vi "SwitchingHTTPCameraResponder.vi"(9 "Switched Camera Name":string, 10 "parameters":T1(array[cluster]), 11 "connection ID":refnum<k5>) -> ()   [LabVIEW 2017, in "ArgosLib.lvlib"]
doc: "This VI is launched each time a new client camera connection is requested. The connection will remain open until closed by the client or because of errors with the camera. Parameters are name/lvalue pairs that have been parsed from a URL request. Supported parameters are name, fps, resolution, compression, exposure, brightness, whitebalance, sharpness, and colorlevel.\n\nThe first four parameters are filled with defaults if not provided, but the latter four are only set if provided."
uses:
  <vilib>/Rock Robotics/SystemInterfaces/NetworkCommunication/NetComm_UsageReport_ResourceType.ctl
  <vilib>/Rock Robotics/WPI/Camera/WPI_CameraImageSize.ctl
  PowerUpSrc/Global_Var-RefNum/SwitchedCameraData.vi
  <vilib>/Utility/error.llb/Error Cluster From Error Code.vi
  <vilib>/ErrorRing/Error Ring.xnode
  ArgosLib.lvlib
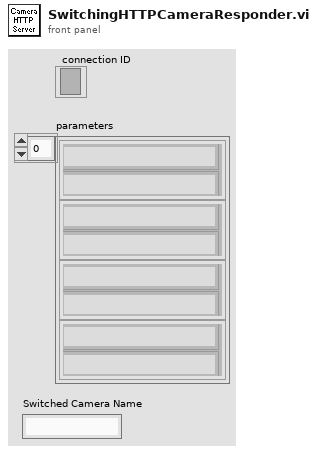
[diagram p1: front panel]
types:
  T1 = cluster{"token string":string, "token string 2":string}[]
  T2 = typedef "Image Type" = u32
  T3 = cluster{"White Balance":string, "Brightness":i32, "Sharpness":i32, "Saturation":i32, "Exposure":string}
  T4 = cluster{"Camera Name":string, "Size":string, "Frame Rate":i32, "Compression":i32}
  T5 = typedef "NetComm_UsageReport_ResourceType.ctl" = enum8{"Controller", "Module", "Language", "CANPlugin", "Accelerometer", "ADXL345", "AnalogChannel", "AnalogTrigger", "AnalogTriggerOutput", "CANJaguar", "Compressor", "Counter", "Dashboard", "DigitalInput", "DigitalOutput", "DriverStationCIO", "DriverStationEIO", "DriverStationLCD", "Encoder", "GearTooth", "Gyro", "I2C", "Framework", "Jaguar", "Joystick", "Kinect", "KinectStick", "PIDController", "Preferences", "PWM", "Relay", "RobotDrive", "SerialPort", "Servo", "Solenoid", "SPI", "Task", "Ultrasonic", "Victor", "Button", "Command", "AxisCamera", "PCVideoServer", "SmartDashboard", "Talon", "HiTechnicColorSensor", "HiTechnicAccel", "HiTechnicCompass", "SRF08", "AnalogOutput", "Victor SP", "Talon SRX", "CAN Talon SRX", "ADXL362 Accel", "ADXRS450 Gyro", "Rev SPARK", "Mindsensors SD540", "Digital Filter", "ADIS16448", "PDP", "PCM", "PigeonIMU", "Nidec Brushless", "CTRE CANifier", "CTRE Future 0", "CTRE Future 1", "CTRE Future 2", "CTRE Future 3", "CTRE Future 4", "CTRE Future 5", "CTRE Future 6"}
  T6 = cluster{"White Balance":bool, "Brightness":bool, "Sharpness":bool, "Saturation":bool, "Exposure":bool}
  T7 = typedef "IMAQ Image.ctl" = refnum<image>
  T8 = typedef "WPI_CameraImageSize.ctl" = enum16{"640x480", "320x240", "160x120", "Custom"}
  T9 = enum16{"Update Mode", "Get Image", "Get Image Data"}
  T10 = typedef "WPI_CameraDevRef.ctl" = cluster{"Camera Address":string, "CameraStatus":errorcluster}
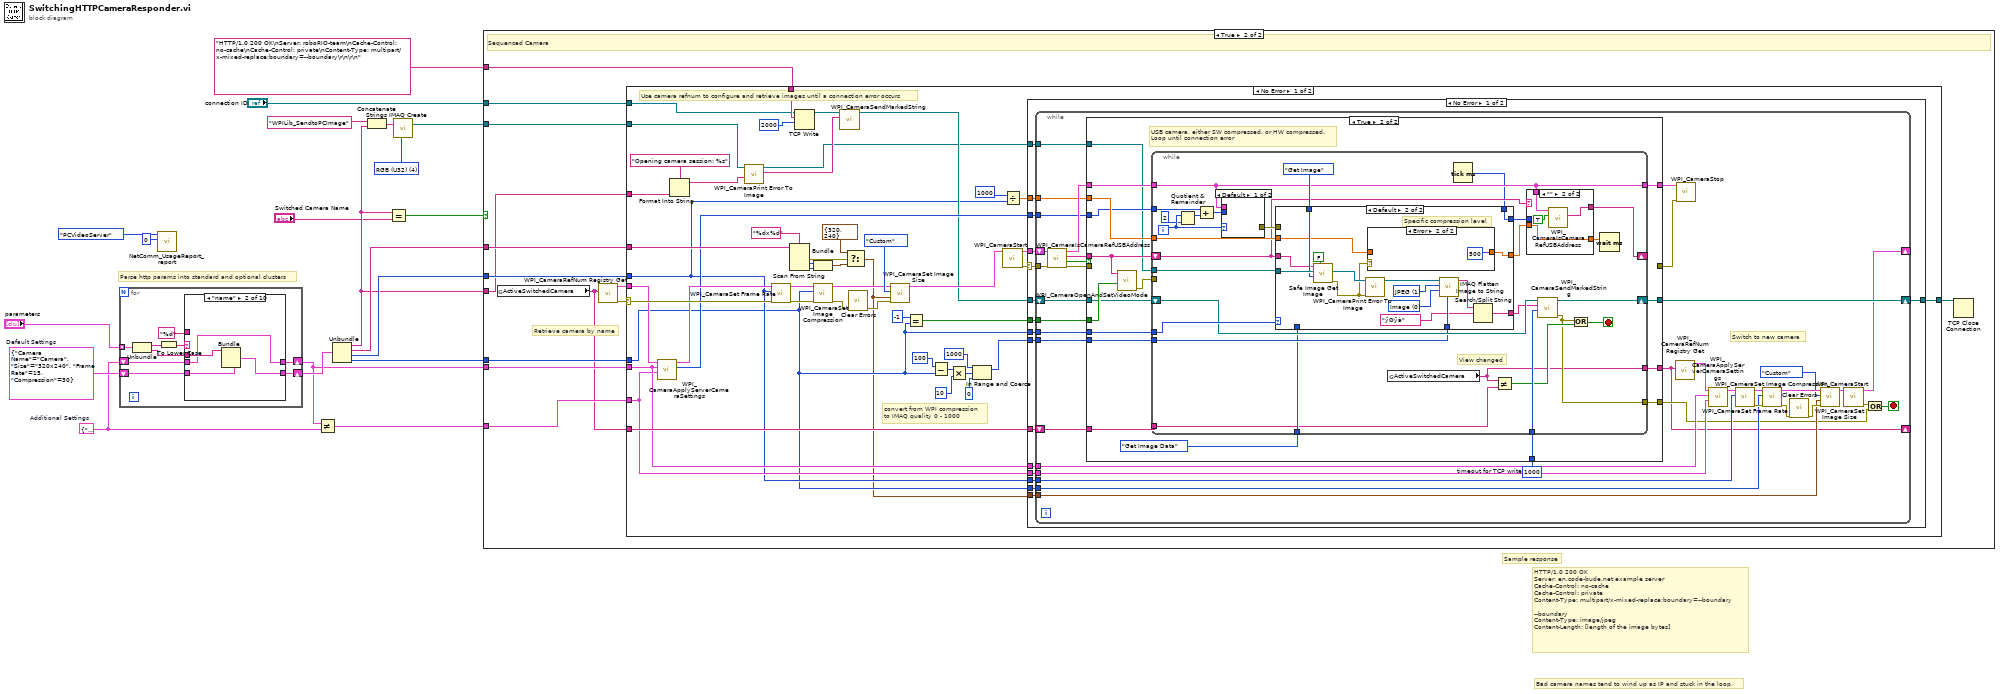
[diagram p0: block diagram]
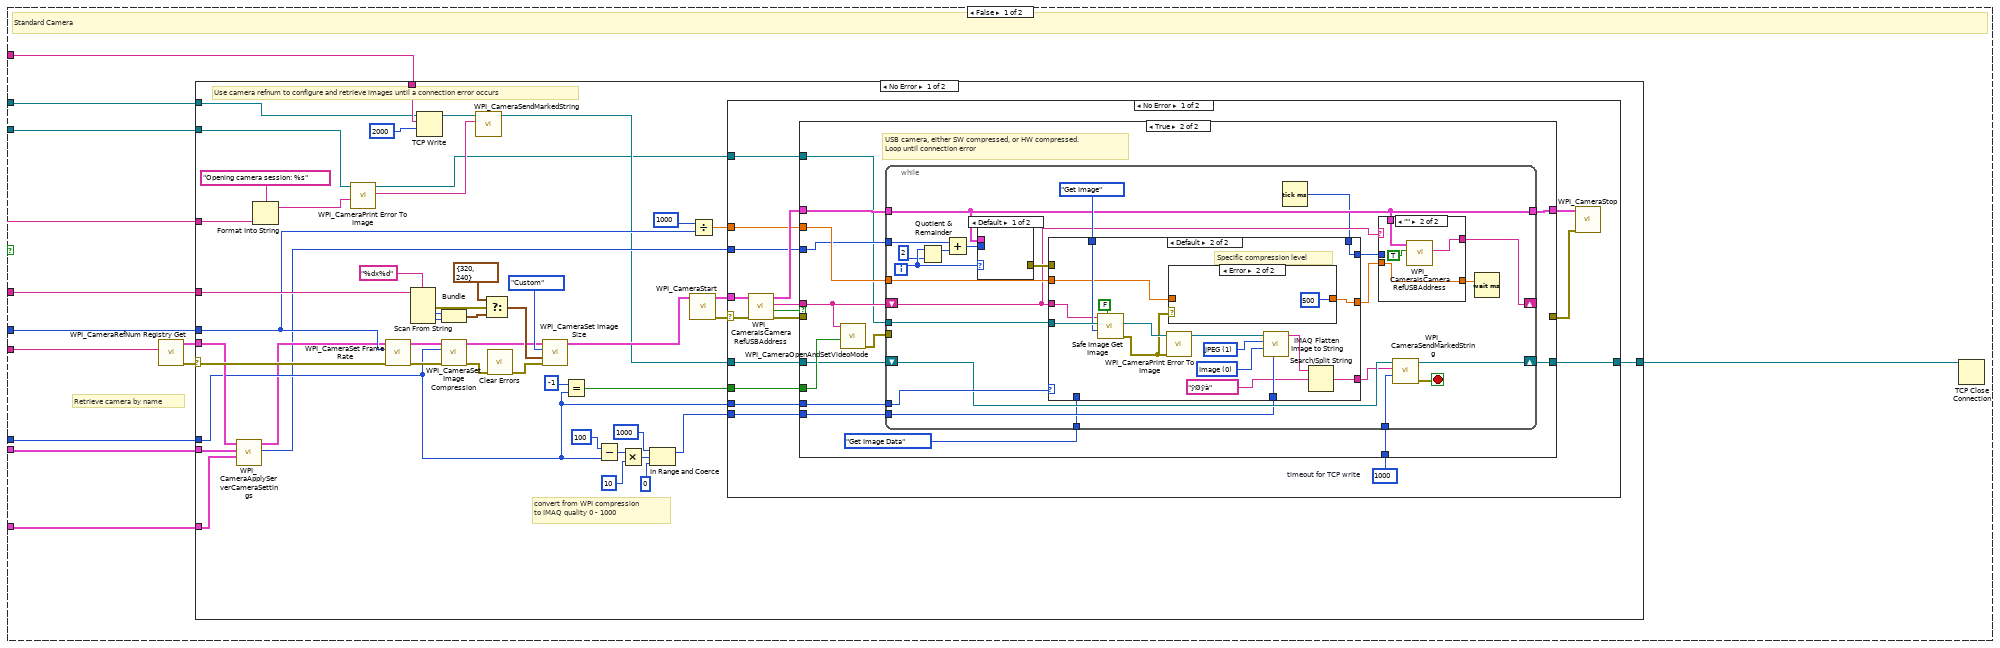
[diagram p2: hidden frame]
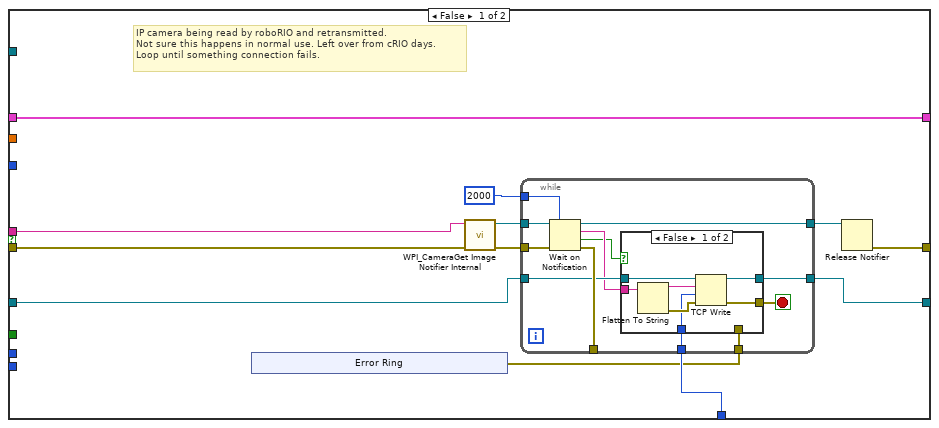
[diagram p3: hidden frame]
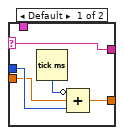
[diagram p5: hidden frame]
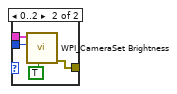
[diagram p6: hidden frame]
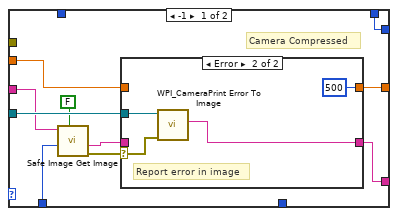
[diagram p7: hidden frame]
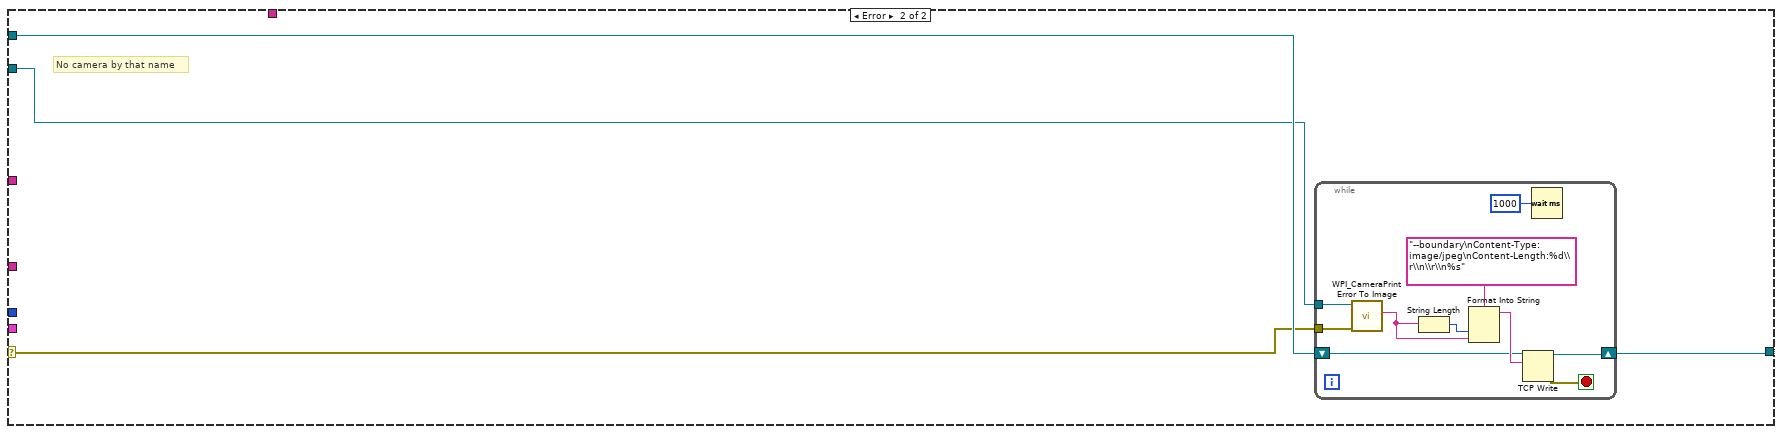
[diagram p11: hidden frame]
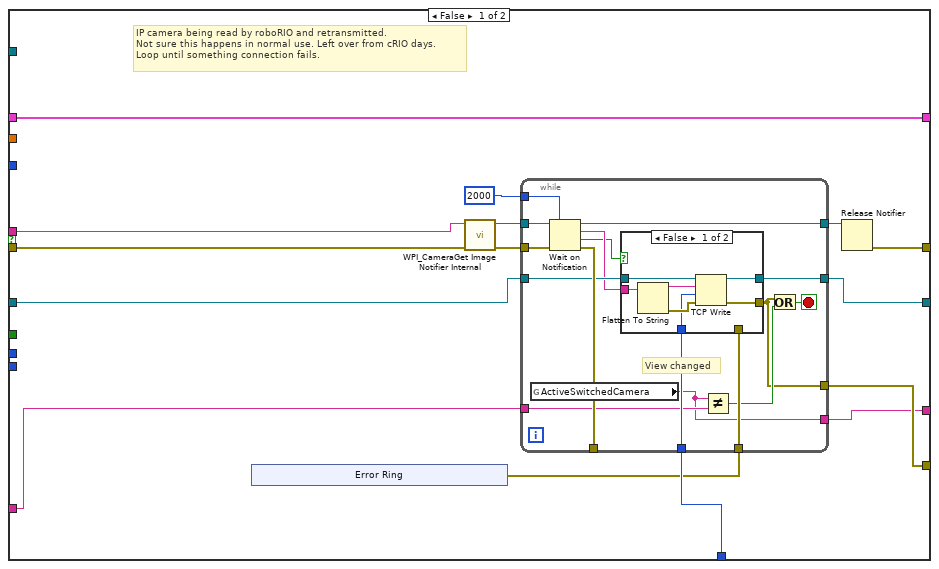
[diagram p12: hidden frame]
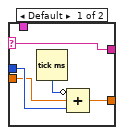
[diagram p14: hidden frame]
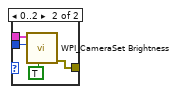
[diagram p15: hidden frame]
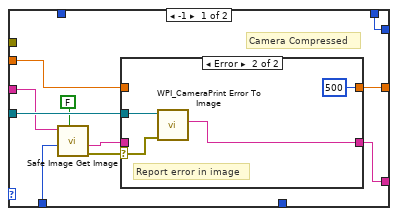
[diagram p16: hidden frame]
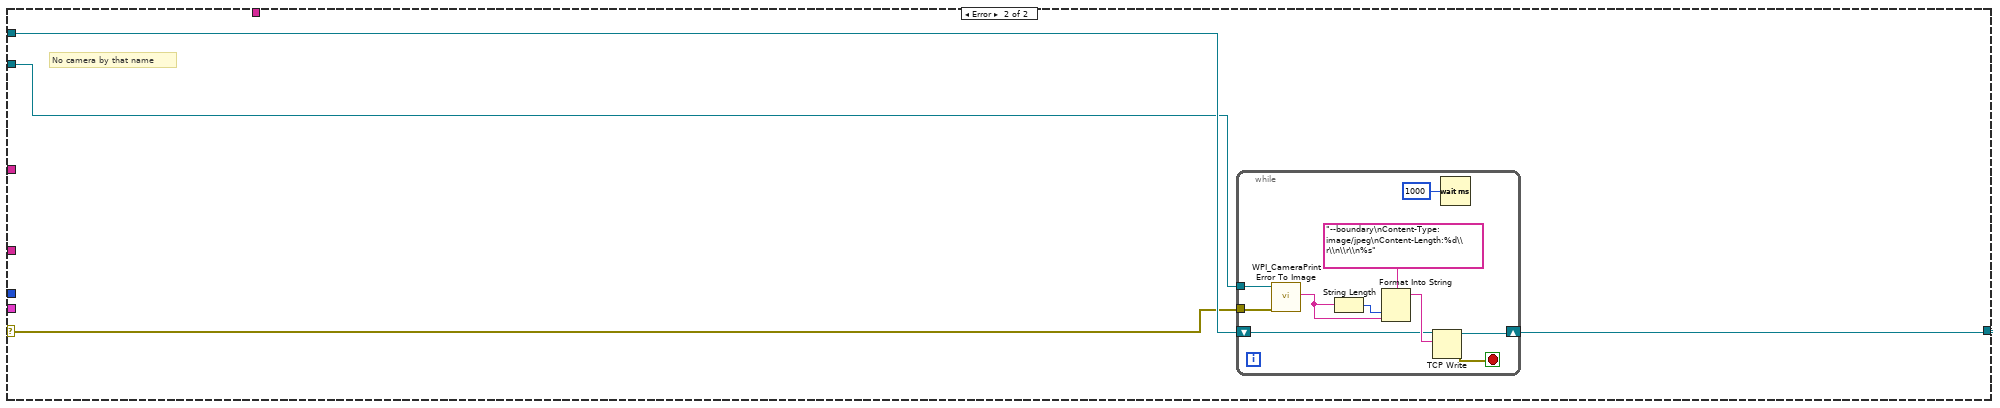
[diagram p20: hidden frame]
diagram:
  w6 = T2 4 items=["Grayscale (U8)", "Grayscale (I16)", "Grayscale (SGL)", "Complex (CSG)", "RGB (U32)", "HSL (U32)", "RGB (U64)", "Grayscale (U16)"] ("Image Type")
  w13 = T3 {"White Balance"="", "Brightness"=-1, "Sharpness"=-1, "Saturation"=-1, "Exposure"=""}  # Additional Settings
  w18 = T4 {"Camera Name"="Camera", "Size"="320x240", "Frame Rate"=15, "Compression"=30}  # Default Settings
  # "Sample response"
  # "HTTP/1.0 200 OK\nServer: en.code-bude.net example server\nCache-Control: no-cache\nCache-Control: private\nContent-Type: multipart/x-mixed-replace;boundary=--boundary\n \n--boundary\nContent-Type: image/jpeg\nContent-Length: [length of the image bytes]"
  # "Parse http params into standard and optional clusters"
  # "Bad camera names tend to wind up as IP and stuck in the loop."
  n1 = for {
    tunnel: "parameters" -> [w29] mode=indexing
    shift-right: [w24] -> w16
    shift-left: w18 -> [w26]
    shift-right: [w21] -> w11
    shift-left: w13 -> [w22]
    n2 = Unbundle(w29) -> ("token string"=w28:string, "token string 2"=w25:string)
    n3 = To Lower Case(string=w28) -> (all lower case string=w27:string)
    n4 = case shown="\"name\"" w27 {
      tunnel: w26 -> [w31 w35 w41 w45 w51 w55 w59 w65 w71 w77]
      tunnel: w25 -> [_ w34 w39 w43 w49 w53 w56 w61 w67 w73]
      tunnel: [w31 w33 w40 w44 w50 w55 w59 w65 w71 w77] -> w24
      tunnel: "%d" -> [_ _ w38 _ w47 _ _ w62 w68 w74]
      tunnel: w22 -> [w30 w32 w36 w42 w46 w54 w58 w64 w70 w76]
      tunnel: [w30 w32 w36 w42 w46 w52 w57 w63 w69 w75] -> w21
      frame Default {
      }
      frame "name" {
        n5 = Bundle(cluster=w35, "Camera Name"=w34) -> (w33:T4)  [unwired: 3 in]
      }
      frame "fps" {
        n6 = Scan From String(format string=w38, input string=w39) -> (output 1=w37:i32)  [unwired: 3 in, 3 out]
        n7 = Bundle(cluster=w41, "Frame Rate"=w37) -> (w40:T4)  [unwired: 3 in]
      }
      frame "resolution" {
        n8 = Bundle(cluster=w45, "Size"=w43) -> (w44:T4)  [unwired: 3 in]
      }
      frame "compression" {
        n9 = Scan From String(format string=w47, input string=w49) -> (output 1=w48:i32)  [unwired: 3 in, 3 out]
        n10 = Bundle(cluster=w51, "Compression"=w48) -> (w50:T4)  [unwired: 3 in]
      }
      frame "whitebalance" {
        n11 = Bundle(cluster=w54, "White Balance"=w53) -> (w52:T3)  [unwired: 4 in]
      }
      frame "exposure" {
        n12 = Bundle(cluster=w58, "Exposure"=w56) -> (w57:T3)  [unwired: 4 in]
      }
      frame "brightness" {
        n13 = Scan From String(format string=w62, input string=w61) -> (output 1=w60:i32)  [unwired: 3 in, 3 out]
        n14 = Bundle(cluster=w64, "Brightness"=w60) -> (w63:T3)  [unwired: 4 in]
      }
      frame "sharpness" {
        n15 = Scan From String(format string=w68, input string=w67) -> (output 1=w66:i32)  [unwired: 3 in, 3 out]
        n16 = Bundle(cluster=w70, "Sharpness"=w66) -> (w69:T3)  [unwired: 4 in]
      }
      frame "colorlevel" {
        n17 = Scan From String(format string=w74, input string=w73) -> (output 1=w72:i32)  [unwired: 3 in, 3 out]
        n18 = Bundle(cluster=w76, "Saturation"=w72) -> (w75:T3)  [unwired: 4 in]
      }
    }
  }
  n19 = call <vilib>:"NetComm_UsageReport_report.vi"("Instance Number"=u8 0, "Resource Type"=NetComm_UsageReport_ResourceType."PCVideoServer") -> ()  [unwired: 10 in]
  n20 = Not Equal?(x=w11, y=w13) -> (x != y?=w12:T6)
  n21 = Unbundle(w16) -> ("Camera Name"=w3:string, "Size"=w17:string, "Frame Rate"=w9:i32, "Compression"=w10:i32)
  n22 = Concatenate Strings("WPILib_SendtoPCImage", w3) -> (w5:string)
  n23 = Equal?(x=w3, y="Switched Camera Name") -> (x = y?=w1:bool)
  n24 = call "IMAQ Create"("Image Name"=w5, "Image Type"=w6) -> ("New Image"=w7:T7)  [unwired: 3 in, 1 out]
  n25 = case shown="True" w1 {
    tunnel: w17 -> [w87 w302]
    tunnel: w12 -> [w86 w301]
    tunnel: w11 -> [w85 w300]
    tunnel: w10 -> [w84 w299]
    tunnel: w9 -> [w83 w298]
    tunnel: "connection ID" -> [w82 w297]
    tunnel: w7 -> [w80 w295]
    tunnel: w3 -> [w79 w294]
    tunnel: "HTTP/1.0 200 OK\nServer: roboRIO-team\nCache-Control: no-cache\nCache-Control: private\nContent-Type: multipart/x-mixed-replace;boundary=--boundary\r\n\r\n" ("regular expression") -> [w78 w293]
    frame False {
      # "Retrieve camera by name"
      # "Standard Camera"
      n26 = call <vilib>:"WPI_CameraRefNum Registry Get.vi"("refnum name"=w79) -> ("error out"=w81:errorcluster, "CameraDevRef"=w88:T10)  [unwired: 9 in]
      n27 = case shown="No Error" w81 {
        selector: w81 -> [w113 w279]
        tunnel: [w137 w280] -> w89
        tunnel: w88 -> [w105 _]
        tunnel: w87 -> [w124 _]
        tunnel: w86 -> [w115 _]
        tunnel: w85 -> [w114 _]
        tunnel: w84 -> [w104 _]
        tunnel: w83 -> [w112 _]
        tunnel: w82 -> [w92 w281]
        tunnel: w80 -> [w97 w278]
        tunnel: w79 -> [w99 _]
        tunnel: w78 -> [w93 _]
        frame No Error {
          # "Use camera refnum to configure and retrieve images until a connection error occurs"
          # "convert from WPI compression\nto IMAQ quality 0 - 1000"
          n28 = call <vilib>:"WPI_CameraApplyServerCameraSettings.vi"("Unique"=w115, "Additional Settings"=w114, "CameraDevRef"=w105) -> ("Brightness"=w102:i32, "CameraDevRef Out"=w103:T10)  [unwired: 7 in]
          n29 = Format Into String(format string="Opening camera session: %s", w99) -> (resulting string=w95:string)  [unwired: 2 in, 1 out]
          n30 = call <vilib>:"WPI_CameraPrint Error To Image.vi"("String"=w95, "Image"=w97) -> ("flattened error string"=w101:string, "Image out"=w96:T7)  [unwired: 8 in]
          n31 = call <vilib>:"WPI_CameraSet Frame Rate.vi"("error in (no error)"=w113, "Frame Rate (fps)"=w112, "CameraDevRef"=w103) -> ("error out"=w109:errorcluster, "CameraDevRef Out"=w111:T10)  [unwired: 7 in]
          n32 = Scan From String(format string="%dx%d", input string=w124) -> (error out=w119:errorcluster, output 1=w122:i32, output 2=w121:i32)  [unwired: 4 in, 2 out]
          n33 = TCP Write(connection ID=w92, data in=w93, 9:2000) -> (connection ID out=w91:refnum<k5>)  [unwired: 1 in, 2 out]
          n34 = Bundle(w122, w121) -> (w118:cluster{i32, i32})  [unwired: 1 in]
          n35 = call <vilib>:"WPI_CameraSet Image Compression.vi"("error in (no error)"=w109, "Compression"=w104, "CameraDevRef"=w111) -> ("error out"=w108:errorcluster, "CameraDevRef Out"=w110:T10)  [unwired: 7 in]
          n36 = call <vilib>:"WPI_CameraSendMarkedString.vi"("Data String"=w101, "TCP Network Connection in"=w91) -> ("TCP Network Connection out"=w100:refnum<k5>)  [unwired: 8 in, 1 out]
          n37 = Select(t=cluster{i32, i32} {320, 240} ("s? t:f"), s=w119, f=w118) -> (s? t:f=w117:cluster{i32, i32})
          n38 = call <vilib>:"Clear Errors.vi"("error in (no error)"=w108) -> ("error out"=w107:errorcluster)  [unwired: 5 in, 1 out]
          n39 = call <vilib>:"WPI_CameraSet Image Size.vi"("error in (no error)"=w107, "Size W,H (pix)"=w117, "Image Size"=WPI_CameraImageSize."Custom", "CameraDevRef"=w110) -> ("CameraDevRef Out"=w106:T10)  [unwired: 6 in, 1 out]
          n40 = Equal?(x=-1, y=w104) -> (x = y?=w125:bool)
          n41 = Subtract(x=100, y=w104) -> (x-y=w129:i32)
          n42 = Multiply(x=w129, y=10) -> (x*y=w131:i32)
          n43 = In Range and Coerce(upper limit=1000, x=w131, lower limit=0) -> (coerced(x)=w127:i32)  [unwired: 1 out]
          n44 = call <vilib>:"WPI_CameraStart.vi"("CameraDevRef"=w106) -> ("error out"=w90:errorcluster, "CameraDevRef"=w136:T10)  [unwired: 1 in, 8 out]
          n45 = Divide(x=u16 1000 ("port"), y=w112) -> (x/y=w134:dbl)
          n46 = case shown="No Error" w90 {
            selector: w90 -> [w138 _]
            tunnel: [w154 w277] -> w137
            tunnel: w136 -> [w149 _]
            tunnel: w134 -> [w147 _]
            tunnel: w127 -> [w146 _]
            tunnel: w125 -> [w145 _]
            tunnel: w104 -> [w142 _]
            tunnel: w102 -> [w141 _]
            tunnel: w100 -> [w140 w277]
            tunnel: w96 -> [w139 _]
            frame No Error {
              w143 = 1000  # timeout for TCP write
              n47 = call <vilib>:"WPI_CameraIsCameraRefUSBAddress.vi"("error in (no error)"=w138, "CameraDevRef"=w149) -> ("error out"=w144:errorcluster, "USB?"=w150:bool, "Camera Address Out"=w151:string, "CameraDevRef out"=w148:T10)  [unwired: 6 in]
              n48 = case shown="True" w150 {
                tunnel: w140 -> [w166 w192]
                tunnel: [w165 w205] -> w154
                tunnel: w144 -> [w164 _]
                tunnel: w151 -> [w162 w201]
                tunnel: [w156 w203] -> w153
                tunnel: w148 -> [w156 w204]
                tunnel: [w160 _] -> w152
                tunnel: w146 -> [_ w198]
                tunnel: w147 -> [_ w196]
                tunnel: w142 -> [_ w202]
                tunnel: w145 -> [_ w200]
                tunnel: w143 -> [w158 w199]
                tunnel: w141 -> [_ w194]
                tunnel: w139 -> [_ w193]
                frame False {
                  # "IP camera being read by roboRIO and retransmitted.\nNot sure this happens in normal use. Left over from cRIO days.\nLoop until something connection fails."
                  n49 = xnode "Error Ring"() -> ("error out"=w155:errorcluster)
                  n50 = call <vilib>:"WPI_CameraGet Image Notifier Internal.vi"("error in (no error)"=w164, "Camera Address"=w162) -> ("error out"=w163:errorcluster, "Image Notifier"=w161:refnum<notifier>)  [unwired: 8 out]
                  n51 = while {
                    tunnel: w163 -> [w182]
                    tunnel: w166 -> [w177]
                    tunnel: [w180] -> _
                    tunnel: [w176] -> w165
                    tunnel: w161 -> [w181]
                    tunnel: [w179] -> w159
                    tunnel: w158 -> [w178]
                    tunnel: w155 -> [w173]
                    tunnel: 2000 ("Timeout in ms (-1)") -> [w172]
                    stop <- w171 stop-if-true
                    n52 = Wait on Notification(notifier=w181, timeout in ms (-1)=w172, error in (no error)=w182) -> (notifier out=w179:refnum<notifier>, notification=w175:string, timed out?=w174:bool, error out=w180:errorcluster)  [unwired: 1 out]
                    n53 = case shown="False" w174 {
                      tunnel: [w187 w190] -> w171
                      tunnel: w178 -> [w186 _]
                      tunnel: w177 -> [w185 w191]
                      tunnel: [w183 w191] -> w176
                      tunnel: w175 -> [w184 _]
                      tunnel: w173 -> [_ w190]
                      frame False {
                        n54 = Flatten To String(anything=w184) -> (data string=w189:string, error out=w188:errorcluster)  [unwired: 1 in, 3 out]
                        n55 = TCP Write(connection ID=w185, data in=w189, error in (no error)=w188, 9:w186) -> (connection ID out=w183:refnum<k5>, error out=w187:errorcluster)  [unwired: 1 out]
                      }
                      frame True {
                      }
                    }
                  }
                  n56 = Release Notifier(notifier=w159) -> (error out=w160:errorcluster)  [unwired: 1 in, 3 out]
                }
                frame True {
                  # "USB camera, either SW compressed, or HW compressed.\nLoop until connection error"
                  n57 = call <vilib>:"WPI_CameraOpenAndSetVideoMode.vi"("USB JPEG"=w200, "Camera Address"=w201) -> ("error out"=w197:errorcluster)  [unwired: 9 in]
                  n58 = while {
                    shift-right: [w222] -> w205
                    shift-left: w192 -> [w227]
                    tunnel: [w212] -> w203
                    tunnel: w204 -> [w212]
                    tunnel: w202 -> [w229]
                    tunnel: w199 -> [w226]
                    tunnel: w198 -> [w225]
                    tunnel: w197 -> [_]
                    tunnel: w196 -> [w221]
                    tunnel: T9."Get Image Data" ("Operation") -> [w220]
                    tunnel: w194 -> [w218]
                    shift-right: [w213] -> _
                    shift-left: w201 -> [w211]
                    tunnel: w193 -> [w210]
                    i -> [w216]
                    stop <- w223 stop-if-true
                    n59 = Quotient & Remainder(x=w216, y=u16 2 ("port")) -> (x-y*floor(x/y)=w217:i32)  [unwired: 1 out]
                    n60 = Add(x=w218, y=w217) -> (x+y=w215:i32)
                    n61 = case shown="Default" w216 {
                      tunnel: w212 -> [_ w242]
                      tunnel: [_ w241] -> w219
                      tunnel: w215 -> [_ w240]
                      frame Default {
                      }
                      frame 0..2 {
                        n62 = call <vilib>:"WPI_CameraSet Brightness.vi"("Force"=TRUE, "Brightness"=w240, "CameraDevRef"=w242) -> ("error out"=w241:errorcluster)  [unwired: 7 in, 1 out]
                      }
                    }
                    n63 = Tick Count (ms)() -> (millisecond timer value=w207:u32)
                    n64 = case shown="Default" w229 {
                      tunnel: [w250 w269] -> w224
                      tunnel: w211 -> [w244 w261]
                      tunnel: w210 -> [w249 w271]
                      tunnel: w225 -> [_ w272]
                      tunnel: T9."Get Image" ("Operation") -> [_ w270]
                      tunnel: w221 -> [w248 w263]
                      tunnel: [w247 w262] -> w209
                      tunnel: w220 -> [w246 _]
                      tunnel: w219 -> [_ _]
                      tunnel: [w243 w260] -> w208
                      tunnel: w207 -> [w243 w260]
                      frame -1 {
                        # "Camera Compressed"
                        n65 = call <vilib>:"Safe Image Get Image.vi"("Wait"=FALSE ("DB"), "Operation"=w246, "Session In"=w244) -> ("error out"=w252:errorcluster, "Image Data String"=w251:string)  [unwired: 5 in, 2 out]
                        n66 = case shown="Error" w252 {
                          selector: w252 -> [_ w258]
                          tunnel: [w254 w255] -> w250
                          tunnel: w251 -> [w254 _]
                          tunnel: w249 -> [_ w257]
                          tunnel: w248 -> [w253 _]
                          tunnel: [w253 u16 500 ("port")] -> w247
                          frame No Error {
                          }
                          frame Error {
                            # "Report error in image"
                            n67 = call <vilib>:"WPI_CameraPrint Error To Image.vi"("error in (no error)"=w258, "Image"=w257) -> ("flattened error string"=w255:string)  [unwired: 8 in, 1 out]
                          }
                        }
                      }
                      frame Default {
                        w273 = 0 items=["Image", "Image and Vision Info", "Reference to Image"] ("Type of Flatten (Image and Vision Info)")
                        w274 = 1 items=["None", "JPEG", "PACKED BINARY"] ("Compression (None)")
                        # "Specific compression level"
                        n68 = call <vilib>:"Safe Image Get Image.vi"("Wait"=FALSE ("DB"), "Operation"=w270, "Image In"=w271, "Session In"=w261) -> ("error out"=w264:errorcluster, "Image Out"=w265:T7)  [unwired: 4 in, 2 out]
                        n69 = call <vilib>:"WPI_CameraPrint Error To Image.vi"("error in (no error)"=w264, "Image"=w265) -> ("Image out"=w267:T7)  [unwired: 8 in, 1 out]
                        n70 = case shown="Error" w264 {
                          tunnel: w263 -> [w275 _]
                          tunnel: [w275 500] -> w262
                          frame No Error {
                          }
                          frame Error {
                          }
                        }
                        n71 = call "IMAQ Flatten Image to String"("Quality (750)"=w272, "Type of Flatten (Image and Vision Info)"=w273, "Compression (None)"=w274, "Image"=w267) -> ("Data String"=w268:string)  [unwired: 6 in, 1 out]
                        n72 = Search/Split String(string=w268, search string/char (-)="ÿØÿà" ("format string")) -> (match + rest of string=w269:string)  [unwired: 1 in, 2 out]
                      }
                    }
                    n73 = case shown="\"\"" w211 {
                      selector: w211 -> [w234 _]
                      tunnel: w212 -> [_ w238]
                      tunnel: [w234 w237] -> w213
                      tunnel: w209 -> [w231 w235]
                      tunnel: w208 -> [w233 _]
                      tunnel: [w232 w235] -> w206
                      frame Default {
                        n74 = Tick Count (ms)() -> (millisecond timer value=w230:u32)
                        n75 = Compound Arithmetic op=ADD(invert w230, w231, w233) -> (w232:dbl)
                      }
                      frame "" {
                        n76 = call <vilib>:"WPI_CameraIsCameraRefUSBAddress.vi"("Enumerate"=TRUE ("Enumerate?"), "CameraDevRef"=w238) -> ("Camera Address Out"=w237:string)  [unwired: 6 in, 3 out]
                      }
                    }
                    n77 = call <vilib>:"WPI_CameraSendMarkedString.vi"("timeout for TCP write"=w226, "Data String"=w224, "TCP Network Connection in"=w227) -> ("error out"=w223:errorcluster, "TCP Network Connection out"=w222:refnum<k5>)  [unwired: 7 in]
                    n78 = Wait (ms)(milliseconds to wait=w206) -> ()  [unwired: 1 out]
                  }
                }
              }
              n79 = call <vilib>:"WPI_CameraStop.vi"("error in (no error)"=w152, "CameraDevRef"=w153) -> ()  [unwired: 10 out]
            }
            frame Error {
            }
          }
        }
        frame Error {
          # "No camera by that name"
          n80 = while {
            shift-right: [w286] -> w280
            shift-left: w281 -> [w285]
            tunnel: w279 -> [w284]
            tunnel: w278 -> [w283]
            stop <- w291 stop-if-true
            n81 = call <vilib>:"WPI_CameraPrint Error To Image.vi"("error in (no error)"=w284, "Image"=w283) -> ("flattened error string"=w289:string)  [unwired: 8 in, 1 out]
            n82 = String Length(string=w289) -> (length=w290:i32)
            n83 = Format Into String(format string="--boundary\nContent-Type: image/jpeg\nContent-Length:%d\\r\\n\\r\\n%s" ("regular expression"), w290, w289) -> (resulting string=w287:string)  [unwired: 2 in, 1 out]
            n84 = TCP Write(connection ID=w285, data in=w287) -> (connection ID out=w286:refnum<k5>, error out=w291:errorcluster)  [unwired: 2 in, 1 out]
            n85 = Wait (ms)(milliseconds to wait=u32 1000) -> ()  [unwired: 1 out]
          }
        }
      }
      n86 = TCP Close Connection(connection ID=w89) -> ()  [unwired: 1 in, 3 out]
    }
    frame True {
      # "Retrieve camera by name"
      # "Sequenced Camera"
      n87 = global read "SwitchedCameraData.vi" "ActiveSwitchedCamera"() -> (w292:string)
      n88 = call <vilib>:"WPI_CameraRefNum Registry Get.vi"("refnum name"=w292) -> ("error out"=w296:errorcluster, "CameraDevRef"=w303:T10)  [unwired: 9 in]
      n89 = case shown="No Error" w296 {
        selector: w296 -> [w332 w545]
        tunnel: [w353 w546] -> w304
        tunnel: w303 -> [w325 _]
        tunnel: w302 -> [w340 _]
        tunnel: w301 -> [w308 _]
        tunnel: w300 -> [w309 _]
        tunnel: w299 -> [w306 _]
        tunnel: w298 -> [w307 _]
        tunnel: w297 -> [w313 w547]
        tunnel: w295 -> [w318 w544]
        tunnel: w294 -> [w320 _]
        tunnel: w293 -> [w314 _]
        tunnel: w292 -> [w310 _]
        frame No Error {
          # "Use camera refnum to configure and retrieve images until a connection error occurs"
          # "convert from WPI compression\nto IMAQ quality 0 - 1000"
          n90 = call <vilib>:"WPI_CameraApplyServerCameraSettings.vi"("Unique"=w308, "Additional Settings"=w309, "CameraDevRef"=w325) -> ("Brightness"=w323:i32, "CameraDevRef Out"=w324:T10)  [unwired: 7 in]
          n91 = Format Into String(format string="Opening camera session: %s", w320) -> (resulting string=w316:string)  [unwired: 2 in, 1 out]
          n92 = call <vilib>:"WPI_CameraPrint Error To Image.vi"("String"=w316, "Image"=w318) -> ("flattened error string"=w322:string, "Image out"=w317:T7)  [unwired: 8 in]
          n93 = call <vilib>:"WPI_CameraSet Frame Rate.vi"("error in (no error)"=w332, "Frame Rate (fps)"=w307, "CameraDevRef"=w324) -> ("error out"=w329:errorcluster, "CameraDevRef Out"=w331:T10)  [unwired: 7 in]
          n94 = Scan From String(format string="%dx%d", input string=w340) -> (error out=w335:errorcluster, output 1=w338:i32, output 2=w337:i32)  [unwired: 4 in, 2 out]
          n95 = TCP Write(connection ID=w313, data in=w314, 9:2000) -> (connection ID out=w312:refnum<k5>)  [unwired: 1 in, 2 out]
          n96 = Bundle(w338, w337) -> (w334:cluster{i32, i32})  [unwired: 1 in]
          n97 = call <vilib>:"WPI_CameraSet Image Compression.vi"("error in (no error)"=w329, "Compression"=w306, "CameraDevRef"=w331) -> ("error out"=w328:errorcluster, "CameraDevRef Out"=w330:T10)  [unwired: 7 in]
          n98 = call <vilib>:"WPI_CameraSendMarkedString.vi"("Data String"=w322, "TCP Network Connection in"=w312) -> ("TCP Network Connection out"=w321:refnum<k5>)  [unwired: 8 in, 1 out]
          n99 = Select(t=cluster{i32, i32} {320, 240} ("s? t:f"), s=w335, f=w334) -> (s? t:f=w305:cluster{i32, i32})
          n100 = call <vilib>:"Clear Errors.vi"("error in (no error)"=w328) -> ("error out"=w327:errorcluster)  [unwired: 5 in, 1 out]
          n101 = call <vilib>:"WPI_CameraSet Image Size.vi"("error in (no error)"=w327, "Size W,H (pix)"=w305, "Image Size"=WPI_CameraImageSize."Custom", "CameraDevRef"=w330) -> ("CameraDevRef Out"=w326:T10)  [unwired: 6 in, 1 out]
          n102 = Equal?(x=-1, y=w306) -> (x = y?=w341:bool)
          n103 = Subtract(x=100, y=w306) -> (x-y=w345:i32)
          n104 = Multiply(x=w345, y=10) -> (x*y=w347:i32)
          n105 = In Range and Coerce(upper limit=1000, x=w347, lower limit=0) -> (coerced(x)=w343:i32)  [unwired: 1 out]
          n106 = call <vilib>:"WPI_CameraStart.vi"("CameraDevRef"=w326) -> ("error out"=w311:errorcluster, "CameraDevRef"=w352:T10)  [unwired: 1 in, 8 out]
          n107 = Divide(x=u16 1000 ("port"), y=w307) -> (x/y=w350:dbl)
          n108 = case shown="No Error" w311 {
            selector: w311 -> [w360 _]
            tunnel: [w369 w543] -> w353
            tunnel: w352 -> [w368 _]
            tunnel: w350 -> [w367 _]
            tunnel: w343 -> [w366 _]
            tunnel: w341 -> [w365 _]
            tunnel: w306 -> [w364 _]
            tunnel: w323 -> [w363 _]
            tunnel: w321 -> [w362 w543]
            tunnel: w317 -> [w361 _]
            tunnel: w310 -> [w359 _]
            tunnel: w309 -> [w358 _]
            tunnel: w308 -> [w357 _]
            tunnel: w307 -> [w356 _]
            tunnel: w306 -> [w355 _]
            tunnel: w305 -> [w354 _]
            frame No Error {
              n109 = while {
                tunnel: w367 -> [w399]
                tunnel: w366 -> [w398]
                tunnel: w365 -> [w397]
                tunnel: w364 -> [w394]
                tunnel: w363 -> [w393]
                tunnel: w361 -> [w391]
                tunnel: w360 -> [w390]
                shift-right: [w406] -> w369
                shift-left: w362 -> [w392]
                shift-right: [w374] -> _
                shift-left: w368 -> [w401]
                tunnel: w358 -> [w387]
                tunnel: w357 -> [w386]
                tunnel: w356 -> [w384]
                tunnel: w355 -> [w381]
                tunnel: w354 -> [w376]
                shift-right: [w370] -> _
                shift-left: w359 -> [w389]
                stop <- w371 stop-if-true
                w395 = 1000  # timeout for TCP write
                # "Switch to new camera"
                n110 = call <vilib>:"WPI_CameraIsCameraRefUSBAddress.vi"("error in (no error)"=w390, "CameraDevRef"=w401) -> ("error out"=w396:errorcluster, "USB?"=w402:bool, "Camera Address Out"=w403:string, "CameraDevRef out"=w400:T10)  [unwired: 6 in]
                n111 = case shown="True" w402 {
                  tunnel: w392 -> [w421 w454]
                  tunnel: [w420 w467] -> w406
                  tunnel: w396 -> [w419 _]
                  tunnel: w403 -> [w417 w463]
                  tunnel: [w411 w465] -> w405
                  tunnel: w400 -> [w411 w466]
                  tunnel: [w415 _] -> w404
                  tunnel: w398 -> [_ w460]
                  tunnel: w399 -> [_ w458]
                  tunnel: w394 -> [_ w464]
                  tunnel: w397 -> [_ w462]
                  tunnel: w395 -> [w413 w461]
                  tunnel: w393 -> [_ w456]
                  tunnel: w391 -> [_ w455]
                  tunnel: w389 -> [w409 w453]
                  tunnel: [w408 w452] -> w372
                  tunnel: [w407 w451] -> w370
                  frame False {
                    # "IP camera being read by roboRIO and retransmitted.\nNot sure this happens in normal use. Left over from cRIO days.\nLoop until something connection fails."
                    n112 = xnode "Error Ring"() -> ("error out"=w410:errorcluster)
                    n113 = call <vilib>:"WPI_CameraGet Image Notifier Internal.vi"("error in (no error)"=w419, "Camera Address"=w417) -> ("error out"=w418:errorcluster, "Image Notifier"=w416:refnum<notifier>)  [unwired: 8 out]
                    n114 = while {
                      tunnel: w418 -> [w441]
                      tunnel: w421 -> [w436]
                      tunnel: [w439] -> _
                      tunnel: [w435] -> w420
                      tunnel: w416 -> [w440]
                      tunnel: [w438] -> w414
                      tunnel: w413 -> [w437]
                      tunnel: w410 -> [w432]
                      tunnel: 2000 ("Timeout in ms (-1)") -> [w431]
                      tunnel: w409 -> [w430]
                      tunnel: [w427] -> w408
                      tunnel: [w426] -> w407
                      stop <- w429 stop-if-true
                      # "View changed"
                      n115 = global read "SwitchedCameraData.vi" "ActiveSwitchedCamera"() -> (w426:string)
                      n116 = Wait on Notification(notifier=w440, timeout in ms (-1)=w431, error in (no error)=w441) -> (notifier out=w438:refnum<notifier>, notification=w434:string, timed out?=w433:bool, error out=w439:errorcluster)  [unwired: 1 out]
                      n117 = case shown="False" w433 {
                        tunnel: [w446 w449] -> w427
                        tunnel: w437 -> [w445 _]
                        tunnel: w436 -> [w444 w450]
                        tunnel: [w442 w450] -> w435
                        tunnel: w434 -> [w443 _]
                        tunnel: w432 -> [_ w449]
                        frame False {
                          n118 = Flatten To String(anything=w443) -> (data string=w448:string, error out=w447:errorcluster)  [unwired: 1 in, 3 out]
                          n119 = TCP Write(connection ID=w444, data in=w448, error in (no error)=w447, 9:w445) -> (connection ID out=w442:refnum<k5>, error out=w446:errorcluster)  [unwired: 1 out]
                        }
                        frame True {
                        }
                      }
                      n120 = Not Equal?(x=w426, y=w430) -> (x != y?=w428:bool)
                      n121 = Or(x=w427, y=w428) -> (x .or. y?=w429:bool)
                    }
                    n122 = Release Notifier(notifier=w414) -> (error out=w415:errorcluster)  [unwired: 1 in, 3 out]
                  }
                  frame True {
                    # "USB camera, either SW compressed, or HW compressed.\nLoop until connection error"
                    n123 = call <vilib>:"WPI_CameraOpenAndSetVideoMode.vi"("USB JPEG"=w462, "Camera Address"=w463) -> ("error out"=w459:errorcluster)  [unwired: 9 in]
                    n124 = while {
                      shift-right: [w489] -> w467
                      shift-left: w454 -> [w493]
                      tunnel: [w479] -> w465
                      tunnel: w466 -> [w479]
                      tunnel: w464 -> [w495]
                      tunnel: w461 -> [w492]
                      tunnel: w460 -> [w491]
                      tunnel: w459 -> [_]
                      tunnel: w458 -> [w488]
                      tunnel: T9."Get Image Data" ("Operation") -> [w487]
                      tunnel: w456 -> [w485]
                      shift-right: [w480] -> _
                      shift-left: w463 -> [w478]
                      tunnel: w455 -> [w477]
                      tunnel: w453 -> [w472]
                      tunnel: [w469] -> w452
                      tunnel: [w468] -> w451
                      i -> [w483]
                      stop <- w470 stop-if-true
                      # "View changed"
                      n125 = Quotient & Remainder(x=w483, y=u16 2 ("port")) -> (x-y*floor(x/y)=w484:i32)  [unwired: 1 out]
                      n126 = Add(x=w485, y=w484) -> (x+y=w482:i32)
                      n127 = case shown="Default" w483 {
                        tunnel: w479 -> [_ w508]
                        tunnel: [_ w507] -> w486
                        tunnel: w482 -> [_ w506]
                        frame Default {
                        }
                        frame 0..2 {
                          n128 = call <vilib>:"WPI_CameraSet Brightness.vi"("Force"=TRUE, "Brightness"=w506, "CameraDevRef"=w508) -> ("error out"=w507:errorcluster)  [unwired: 7 in, 1 out]
                        }
                      }
                      n129 = global read "SwitchedCameraData.vi" "ActiveSwitchedCamera"() -> (w468:string)
                      n130 = Tick Count (ms)() -> (millisecond timer value=w474:u32)
                      n131 = case shown="Default" w495 {
                        tunnel: [w516 w535] -> w490
                        tunnel: w478 -> [w510 w527]
                        tunnel: w477 -> [w515 w537]
                        tunnel: w491 -> [_ w538]
                        tunnel: T9."Get Image" ("Operation") -> [_ w536]
                        tunnel: w488 -> [w514 w529]
                        tunnel: [w513 w528] -> w476
                        tunnel: w487 -> [w512 _]
                        tunnel: w486 -> [_ _]
                        tunnel: [w509 w526] -> w475
                        tunnel: w474 -> [w509 w526]
                        frame -1 {
                          # "Camera Compressed"
                          n132 = call <vilib>:"Safe Image Get Image.vi"("Wait"=FALSE ("DB"), "Operation"=w512, "Session In"=w510) -> ("error out"=w518:errorcluster, "Image Data String"=w517:string)  [unwired: 5 in, 2 out]
                          n133 = case shown="Error" w518 {
                            selector: w518 -> [_ w524]
                            tunnel: [w520 w521] -> w516
                            tunnel: w517 -> [w520 _]
                            tunnel: w515 -> [_ w523]
                            tunnel: w514 -> [w519 _]
                            tunnel: [w519 u16 500 ("port")] -> w513
                            frame No Error {
                            }
                            frame Error {
                              # "Report error in image"
                              n134 = call <vilib>:"WPI_CameraPrint Error To Image.vi"("error in (no error)"=w524, "Image"=w523) -> ("flattened error string"=w521:string)  [unwired: 8 in, 1 out]
                            }
                          }
                        }
                        frame Default {
                          w539 = 0 items=["Image", "Image and Vision Info", "Reference to Image"] ("Type of Flatten (Image and Vision Info)")
                          w540 = 1 items=["None", "JPEG", "PACKED BINARY"] ("Compression (None)")
                          # "Specific compression level"
                          n135 = call <vilib>:"Safe Image Get Image.vi"("Wait"=FALSE ("DB"), "Operation"=w536, "Image In"=w537, "Session In"=w527) -> ("error out"=w530:errorcluster, "Image Out"=w531:T7)  [unwired: 4 in, 2 out]
                          n136 = call <vilib>:"WPI_CameraPrint Error To Image.vi"("error in (no error)"=w530, "Image"=w531) -> ("Image out"=w533:T7)  [unwired: 8 in, 1 out]
                          n137 = case shown="Error" w530 {
                            tunnel: w529 -> [w541 _]
                            tunnel: [w541 500] -> w528
                            frame No Error {
                            }
                            frame Error {
                            }
                          }
                          n138 = call "IMAQ Flatten Image to String"("Quality (750)"=w538, "Type of Flatten (Image and Vision Info)"=w539, "Compression (None)"=w540, "Image"=w533) -> ("Data String"=w534:string)  [unwired: 6 in, 1 out]
                          n139 = Search/Split String(string=w534, search string/char (-)="ÿØÿà" ("format string")) -> (match + rest of string=w535:string)  [unwired: 1 in, 2 out]
                        }
                      }
                      n140 = Not Equal?(x=w468, y=w472) -> (x != y?=w471:bool)
                      n141 = case shown="\"\"" w478 {
                        selector: w478 -> [w500 _]
                        tunnel: w479 -> [_ w504]
                        tunnel: [w500 w503] -> w480
                        tunnel: w476 -> [w497 w501]
                        tunnel: w475 -> [w499 _]
                        tunnel: [w498 w501] -> w473
                        frame Default {
                          n142 = Tick Count (ms)() -> (millisecond timer value=w496:u32)
                          n143 = Compound Arithmetic op=ADD(invert w496, w497, w499) -> (w498:dbl)
                        }
                        frame "" {
                          n144 = call <vilib>:"WPI_CameraIsCameraRefUSBAddress.vi"("Enumerate"=TRUE ("Enumerate?"), "CameraDevRef"=w504) -> ("Camera Address Out"=w503:string)  [unwired: 6 in, 3 out]
                        }
                      }
                      n145 = call <vilib>:"WPI_CameraSendMarkedString.vi"("timeout for TCP write"=w492, "Data String"=w490, "TCP Network Connection in"=w493) -> ("error out"=w469:errorcluster, "TCP Network Connection out"=w489:refnum<k5>)  [unwired: 7 in]
                      n146 = Or(x=w469, y=w471) -> (x .or. y?=w470:bool)
                      n147 = Wait (ms)(milliseconds to wait=w473) -> ()  [unwired: 1 out]
                    }
                  }
                }
                n148 = call <vilib>:"WPI_CameraRefNum Registry Get.vi"("refnum name"=w370) -> ("CameraDevRef"=w388:T10)  [unwired: 9 in, 1 out]
                n149 = call <vilib>:"WPI_CameraStop.vi"("error in (no error)"=w404, "CameraDevRef"=w405) -> ()  [unwired: 10 out]
                n150 = call <vilib>:"WPI_CameraApplyServerCameraSettings.vi"("Unique"=w386, "Additional Settings"=w387, "CameraDevRef"=w388) -> ("CameraDevRef Out"=w385:T10)  [unwired: 7 in, 1 out]
                n151 = call <vilib>:"WPI_CameraSet Frame Rate.vi"("Frame Rate (fps)"=w384, "CameraDevRef"=w385) -> ("error out"=w382:errorcluster, "CameraDevRef Out"=w383:T10)  [unwired: 8 in]
                n152 = call <vilib>:"WPI_CameraSet Image Compression.vi"("error in (no error)"=w382, "Compression"=w381, "CameraDevRef"=w383) -> ("error out"=w380:errorcluster, "CameraDevRef Out"=w378:T10)  [unwired: 7 in]
                n153 = call <vilib>:"Clear Errors.vi"("error in (no error)"=w380) -> ("error out"=w379:errorcluster)  [unwired: 5 in, 1 out]
                n154 = call <vilib>:"WPI_CameraSet Image Size.vi"("error in (no error)"=w379, "Size W,H (pix)"=w376, "Image Size"=WPI_CameraImageSize."Custom", "CameraDevRef"=w378) -> ("CameraDevRef Out"=w375:T10)  [unwired: 6 in, 1 out]
                n155 = call <vilib>:"WPI_CameraStart.vi"("CameraDevRef"=w375) -> ("error out"=w373:errorcluster, "CameraDevRef"=w374:T10)  [unwired: 1 in, 8 out]
                n156 = Or(x=w373, y=w372) -> (x .or. y?=w371:bool)
              }
            }
            frame Error {
            }
          }
        }
        frame Error {
          # "No camera by that name"
          n157 = while {
            shift-right: [w552] -> w546
            shift-left: w547 -> [w551]
            tunnel: w545 -> [w550]
            tunnel: w544 -> [w549]
            stop <- w557 stop-if-true
            n158 = call <vilib>:"WPI_CameraPrint Error To Image.vi"("error in (no error)"=w550, "Image"=w549) -> ("flattened error string"=w555:string)  [unwired: 8 in, 1 out]
            n159 = String Length(string=w555) -> (length=w556:i32)
            n160 = Format Into String(format string="--boundary\nContent-Type: image/jpeg\nContent-Length:%d\\r\\n\\r\\n%s" ("regular expression"), w556, w555) -> (resulting string=w553:string)  [unwired: 2 in, 1 out]
            n161 = TCP Write(connection ID=w551, data in=w553) -> (connection ID out=w552:refnum<k5>, error out=w557:errorcluster)  [unwired: 2 in, 1 out]
            n162 = Wait (ms)(milliseconds to wait=u32 1000) -> ()  [unwired: 1 out]
          }
        }
      }
      n163 = TCP Close Connection(connection ID=w304) -> ()  [unwired: 1 in, 3 out]
    }
  }
